vi "Read Slide Images.vi"(8 "error in (no error)":errorcluster, 11 "Parse Presentation in":refnum<class "Parse Presentation.lvclass">) -> (0 "error out":errorcluster, 2 "Slide Images":string, 3 "Parse Presentation out":refnum<class "Parse Presentation.lvclass">)   [LabVIEW 2015, in "Parse Presentation.lvclass"]
uses:
  Parse Presentation.lvclass
  Parse Presentation.lvclass/Parse Presentation.ctl
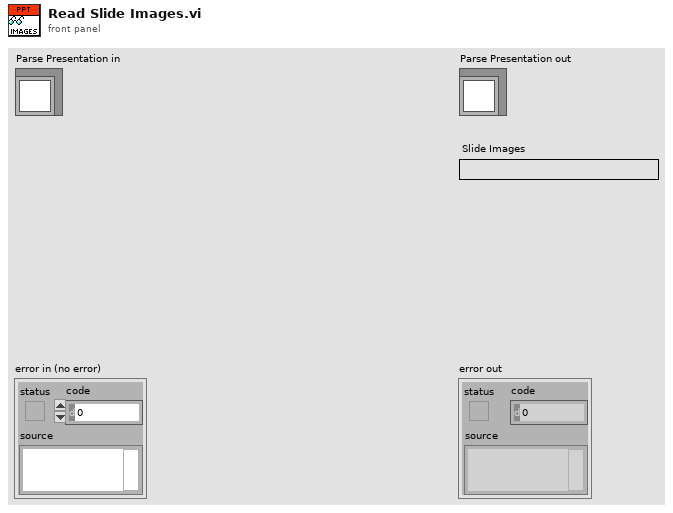
[diagram p1: front panel]
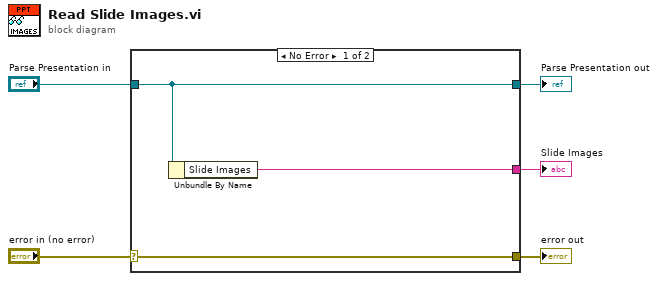
[diagram p0: block diagram]
diagram:
  n1 = case shown="No Error" "error in (no error)" {
    selector: "error in (no error)" -> [w8 w9]
    tunnel: [w8 w9] -> w4
    tunnel: [w7 w10] -> w2
    tunnel: "Parse Presentation in" -> [w7 w10]
    tunnel: [w6 _] -> w1
    frame No Error {
      n2 = Unbundle By Name(w7) -> ("Slide Images"=w6:string)
    }
    frame Error {
    }
  }
  "error out" <- w4
  "Parse Presentation out" <- w2
  "Slide Images" <- w1
